vi "Manual CV paramter_append.vi"(10 "Array":string[][](array[string]), 11 "Path":path) -> (3 "appended array":string[][](array[string]))   [LabVIEW 2009]
doc: "Reads from a spreedsheet file and transposes the data, then appends 2 1 x 1 empty arrays and a 2-D string array. Finally, the VI transposes the new array, returns it, and writes it to the same location as the original spreedsheet array."
uses:
  <vilib>/Utility/file.llb/Write To Spreadsheet File (string).vi
  <vilib>/Utility/file.llb/Read From Spreadsheet File (string).vi
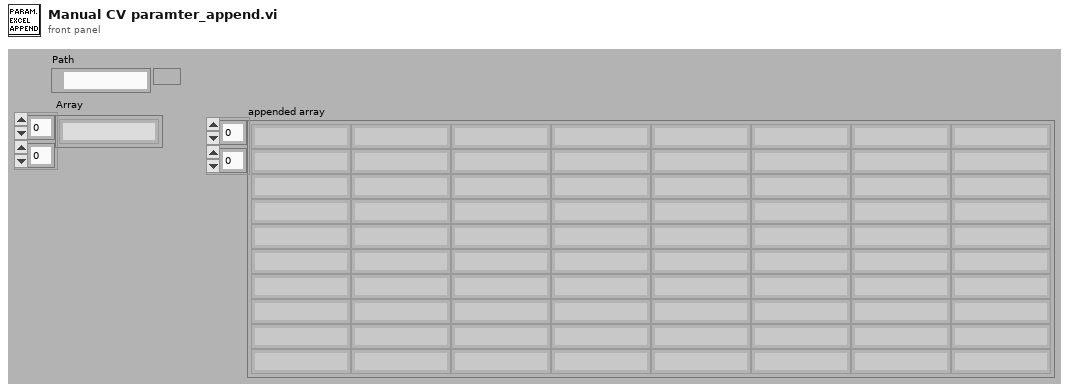
[diagram p1: front panel]
types:
  T1 = enum16{"open", "replace", "create", "open or create", "replace or create", "replace or create with confirmation"}
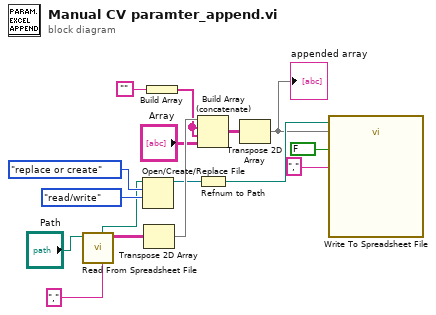
[diagram p0: block diagram]
diagram:
  n1 = call-poly <vilib>:"Read From Spreadsheet File.vi"("delimiter (\\t)"=",", "file path (dialog if empty)"="Path") -> ("all rows"=w16:string[][], "new file path (Not A Path if cancelled)"=w5:path)  [unwired: 5 in, 3 out]
  n2 = Open/Create/Replace File(file path (use dialog)=w5, operation (0:open)=T1."replace or create", access (0:read/write)=enum16{"read/write", "read-only", "write-only"}."read/write") -> (refnum out=w7:refnum<file>)  [unwired: 1 in, 4 out]
  n3 = Transpose 2D Array(2D array=w16) -> (transposed array=w14:string[][])
  n4 = Build Array("") -> (w13:string[])
  n5 = Build Array (concatenate)(w14, w13, w13, "Array") -> (w3:string[][])
  n6 = Refnum to Path(1:w7) -> (0:w4:path)
  n7 = Transpose 2D Array(2D array=w3) -> (transposed array=w2:string[][])
  "appended array" <- w2
  n8 = call-poly <vilib>:"Write To Spreadsheet File.vi"("delimiter (\\t)"=",", "append to file? (new file:F)"=FALSE, "2D data"=w2, "file path (dialog if empty)"=w4) -> ()  [unwired: 3 in, 2 out]
